vi "Regulate Menu.vi"(6 "Run Mode?":bool, 7 "Multiplot Representation In":T1, 8 "error in (no error)":errorcluster, 9 "MenuRef":refnum<k9>, 11 "3D Plot.lvclass in":refnum<class "3D Plot.lvclass">) -> (0 "error out":errorcluster, 1 "Dup MenuRef":refnum<k9>, 3 "3D Plot.lvclass out":refnum<class "3D Plot.lvclass">, 5 "Multiplot Representation Out":T1)   [LabVIEW 2017, in "3D Plot.lvclass"]
uses:
  <vilib>/Math Plots/3D Math Plots/3D Plot/3D Plot/3D Plot.lvclass
  <vilib>/Math Plots/3D Math Plots/3D Plot/3D Plot/Typedef/Multiplot Representation.ctl
  <vilib>/Math Plots/3D Math Plots/3D Plot/3D Plot/Typedef/Plot Representation.ctl
  <vilib>/Math Plots/3D Math Plots/3D Plot/3D Plot/Typedef/Range Clusters.ctl
  <vilib>/Math Plots/3D Math Plots/3D Plot/3D Plot/Typedef/Mesh Data.ctl
  <vilib>/Math Plots/3D Math Plots/3D Plot/3D Plot/3D Plot.lvclass/3D Plot.ctl
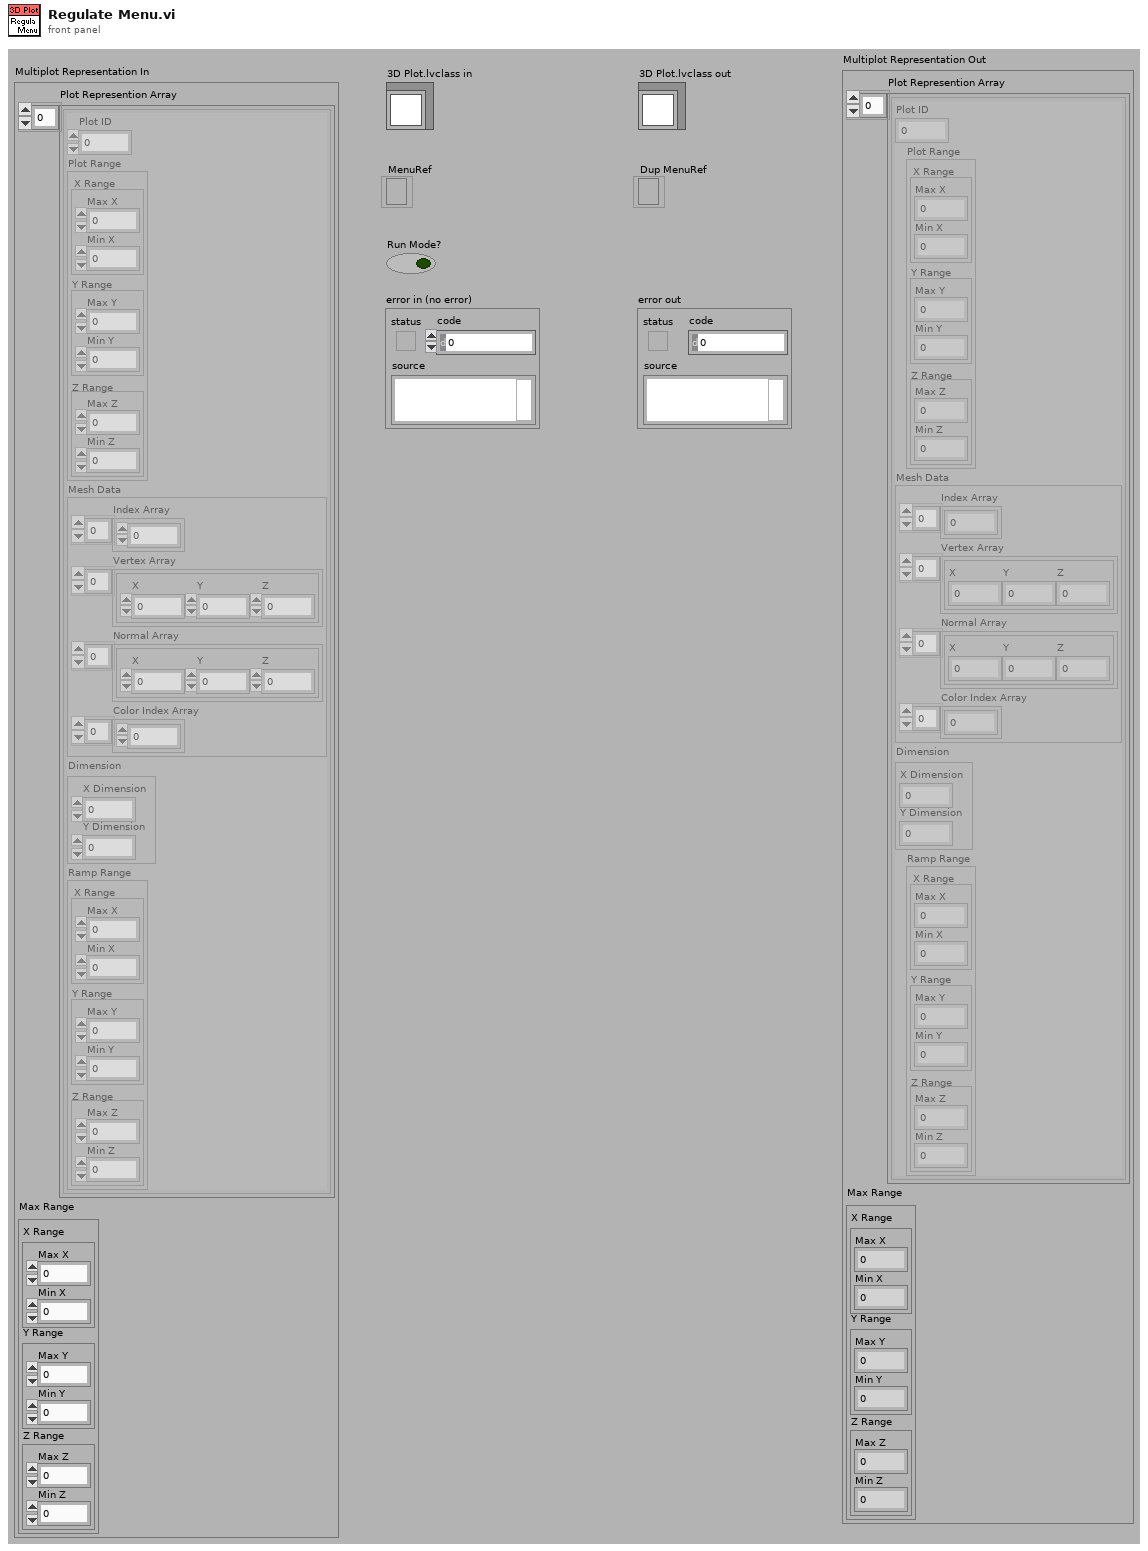
[diagram p1: front panel]
types:
  T1 = typedef "3D Plot.lvclass/Multiplot Representation.ctl" = cluster{"Plot Represention Array":T2[], "Max Range":T3}
  T2 = typedef "3D Plot.lvclass/Plot Representation.ctl" = cluster{"Plot ID":i32, "Plot Range":T3, "Mesh Data":T4, "Dimension":cluster{"X Dimension":i32, "Y Dimension":i32}, "Ramp Range":T3}
  T3 = typedef "3D Plot.lvclass/Range Clusters.ctl" = cluster{"X Range":cluster{"Max X":sgl, "Min X":sgl}, "Y Range":cluster{"Max Y":sgl, "Min Y":sgl}, "Z Range":cluster{"Max Z":sgl, "Min Z":sgl}}
  T4 = typedef "3D Plot.lvclass/Mesh Data.ctl" = cluster{"Index Array":u32[], "Vertex Array":cluster{"X":sgl, "Y":sgl, "Z":sgl}[], "Normal Array":cluster{"X":sgl, "Y":sgl, "Z":sgl}[], "Color Index Array":i32[]}
  T5 = typedef "3D Plot.lvclass/Item Visibility.ctl" = cluster{"Projection Palette":bool, "Color Ramp Palette":bool}
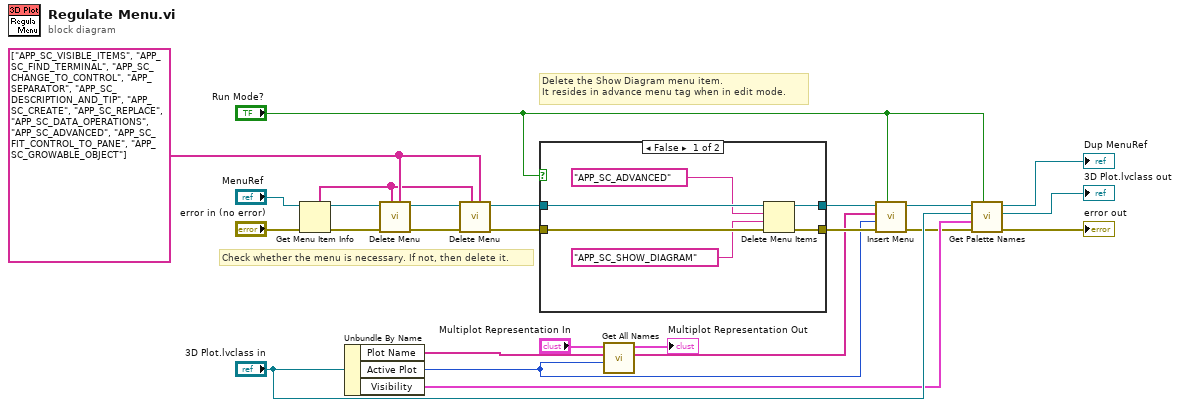
[diagram p0: block diagram]
diagram:
  w21 = string[] ["APP_SC_VISIBLE_ITEMS", "APP_SC_FIND_TERMINAL", "APP_SC_CHANGE_TO_CONTROL", "APP_SEPARATOR", "APP_SC_DESCRIPTION_AND_TIP", "APP_SC_CREATE", "APP_SC_REPLACE", "APP_SC_DATA_OPERATIONS", "APP_SC_ADVANCED", "APP_SC_FIT_CONTROL_TO_PANE", "APP_SC_GROWABLE_OBJECT"] ("submenu tags")
  # "Delete the Show Diagram menu item.\nIt resides in advance menu tag when in edit mode."
  # "Check whether the menu is necessary. If not, then delete it."
  n1 = Get Menu Item Info(8:"error in (no error)", 11:"MenuRef") -> (0:w23:errorcluster, 3:w24:refnum<k9>, 5:w13:string[])  [unwired: 5 out]
  n2 = Unbundle By Name("3D Plot.lvclass in") -> ("Plot Name"=w16:string[], "Active Plot"=w2:i32, "Visibility"=w8:T5)
  n3 = call <vilib>:"Delete Menu.vi"("Submenu Tags Validated"=w21, "Submenu Tags to Check"=w13, "error in (no error)"=w23, "MenuRef"=w24) -> ("error out"=w19:errorcluster, "Dup MenuRef"=w20:refnum<k9>)  [unwired: 6 in]
  n4 = call <vilib>:"Delete Menu.vi"("Submenu Tags Validated"=w21, "Submenu Tags to Check"=w13, "error in (no error)"=w19, "MenuRef"=w20) -> ("error out"=w14:errorcluster, "Dup MenuRef"=w15:refnum<k9>)  [unwired: 6 in]
  n5 = case shown="False" "Run Mode?" {
    tunnel: w15 -> [w31 w33]
    tunnel: w14 -> [w30 w32]
    tunnel: [w26 w32] -> w5
    tunnel: [w27 w33] -> w7
    frame False {
      n6 = Delete Menu Items(6:w30, 7:"APP_SC_SHOW_DIAGRAM" ("menu tag"), 8:"APP_SC_ADVANCED" ("menu tag"), 9:w31) -> (0:w26:errorcluster, 3:w27:refnum<k9>)
    }
    frame True {
    }
  }
  n7 = call <vilib>:"Get All Names.vi"("Active Plot"=w2, "Plot Name In"=w16, "Multiplot Representation In"="Multiplot Representation In") -> ("Plot Name Out"=w3:string[], "Multiplot Representation Out"=→"Multiplot Representation Out":T1)  [unwired: 6 in, 1 out]
  n8 = call <vilib>:"Insert Menu.vi"("Run Mode?"="Run Mode?", "error in (no error)"=w5, "Active Plot ID"=w2, "Plot Names"=w3, "MenuRef"=w7) -> ("error out"=w4:errorcluster, "Dup MenuRef"=w6:refnum<k9>)  [unwired: 1 in, 4 out]
  n9 = call-dynamic "Get Palette Names.vi"("Run Mode?"="Run Mode?", "error in (no error)"=w4, "Visibility"=w8, "3D Plot.lvclass in"="3D Plot.lvclass in", "MenuRef"=w6) -> ("error out"=→"error out":errorcluster, "3D Plot.lvclass out"=→"3D Plot.lvclass out":refnum<class "3D Plot.lvclass">, "Dup MenuRef"=→"Dup MenuRef":refnum<k9>)  [unwired: 4 in]
